vi "finding chrimson rails.vi"() -> ()   [LabVIEW 2014]
uses:
  <vilib>/userdefined/High Color/IMAQdx.ctl
  <vilib>/Utility/file.llb/Write To Spreadsheet File (DBL).vi
  <vilib>/vision/driver/NI_Vision_Acquisition_Software.lvlib
panel:
  in  "Tags":string
  out "Save Directory":path
  in  "Frames before Stimulus":i32
  out "Percent completed":dbl
  in  "Wait between stimuli (seconds)":dbl
  in  "pulse duration (frames)":i32
  in  "GO":bool
  in  "Array":dbl[](array[numeric])
  in  "Trials Per Voltage":i32
  in  "Frames":i32
  out "Error":string
  out "Buffer Number Out":u32
  out "Image":T1(plugin-control)
  in  "stop":bool
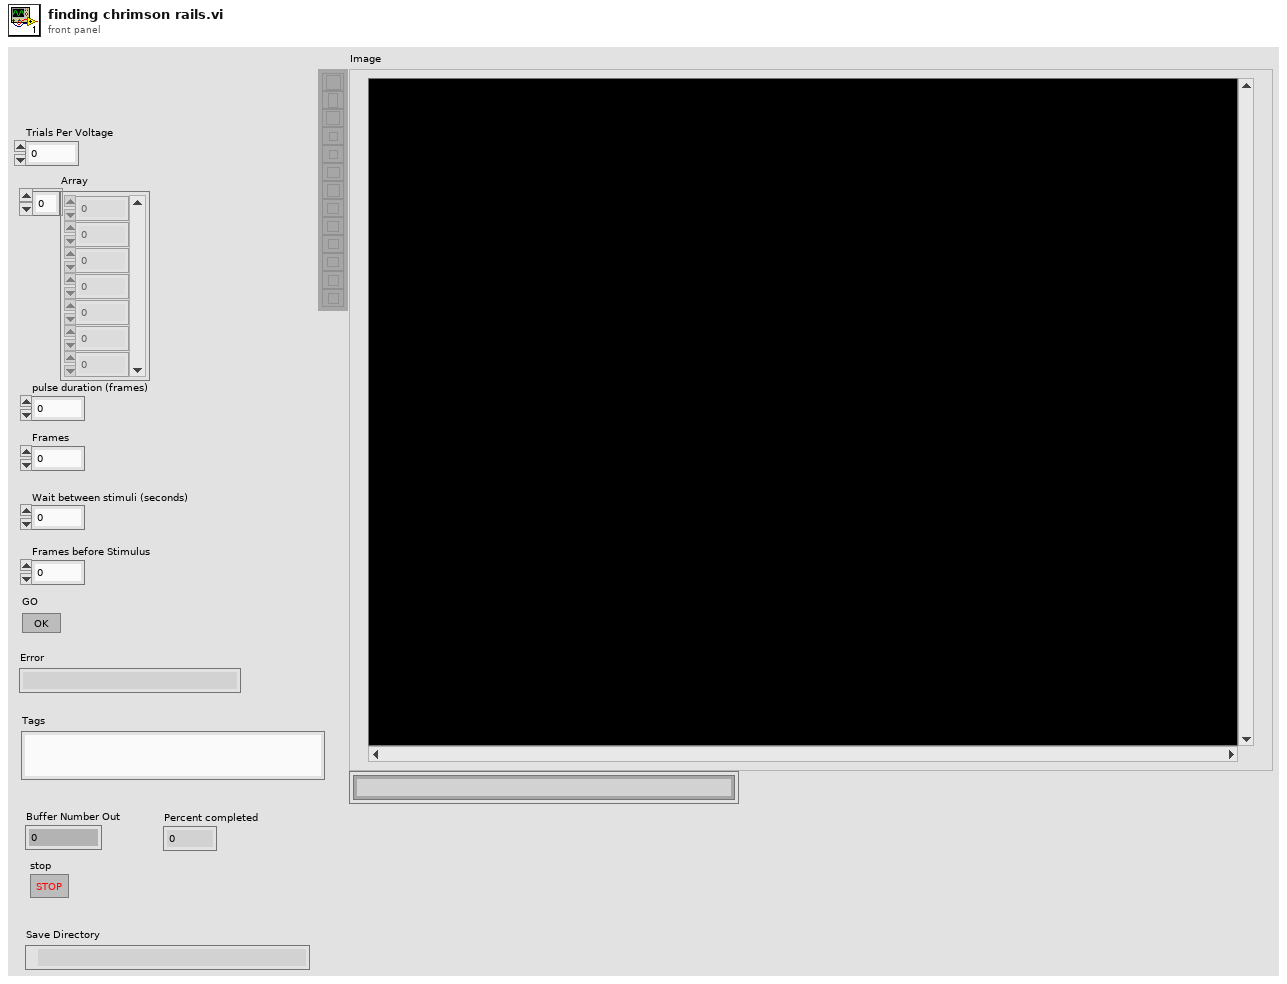
[diagram p1: front panel]
types:
  T1 = typedef "IMAQ Image.ctl" = refnum<image>
  T2 = typedef "IMAQdx.ctl" = refnum<k21>
  T3 = cluster{"Rows Per Strip":i32, "Photometric":i32, "Compression Type":i32}
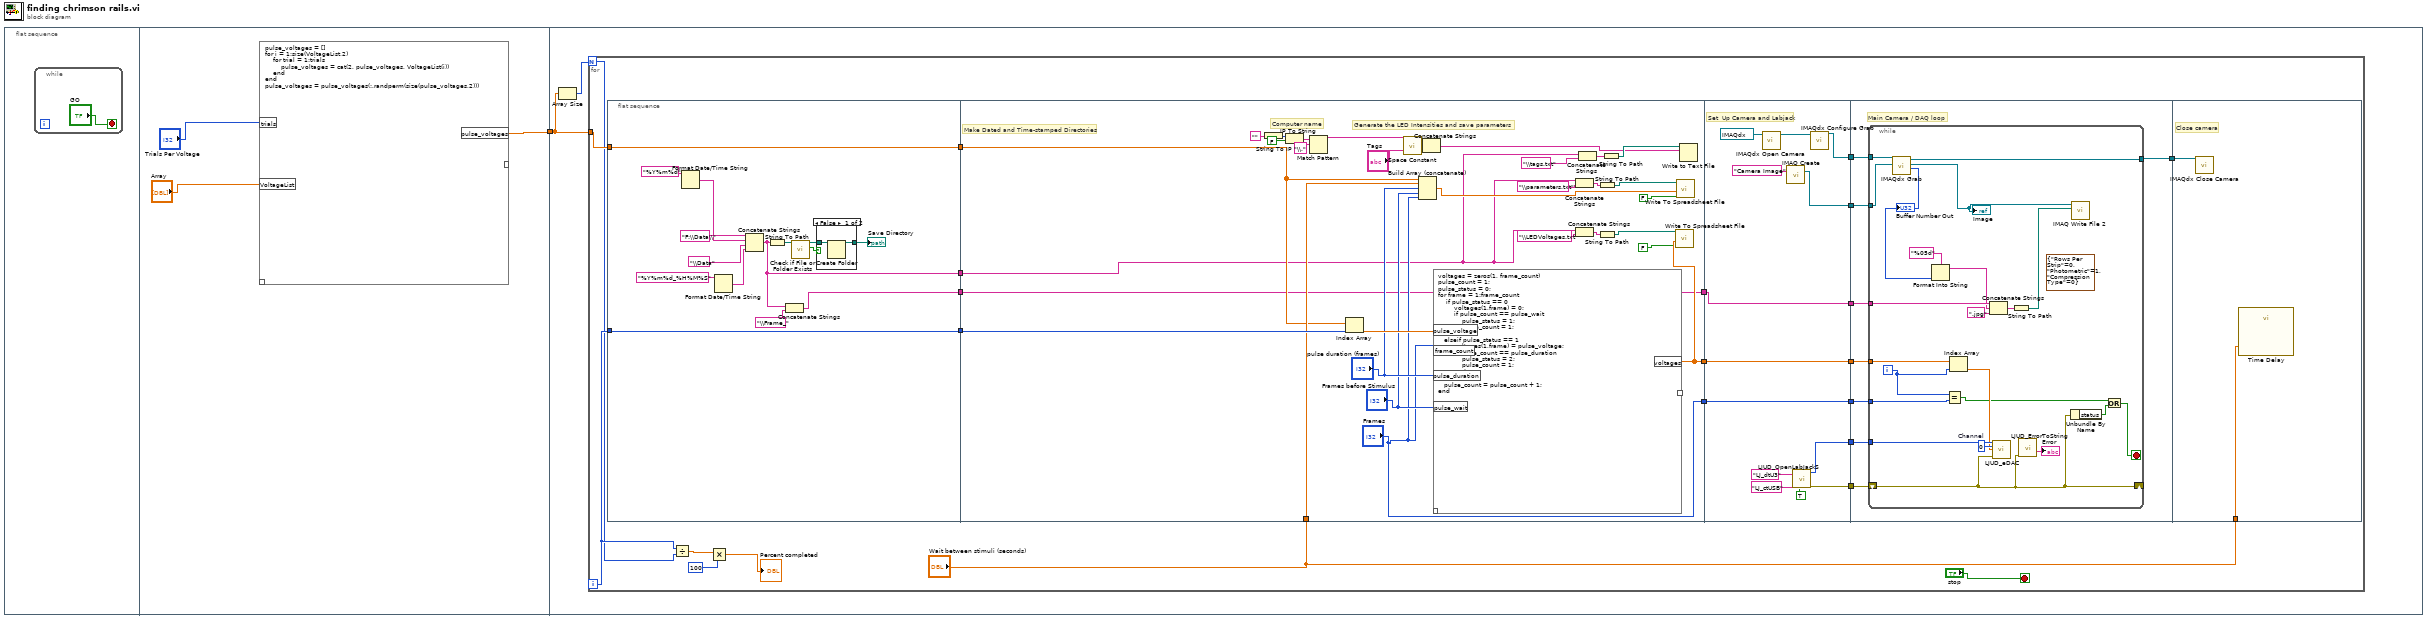
[diagram p0: block diagram]
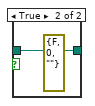
[diagram p2: hidden frame]
diagram:
  n1 = flat-sequence {
    tunnel: [w4] -> w1
    tunnel: w1 -> [w7]
    frame #0 {
      n2 = while {
        stop <- "GO" stop-if-true
      }
    }
    frame #1 {
      n3 = script code="pulse_voltages = []\nfor i = 1:size(VoltageList,2)\n    for trial = 1:trials\n        pulse_voltages = cat(2, pulse_voltages, VoltageList(i))\n    end\nend\npulse_voltages = pulse_voltages(:,randperm(size(pulse_voltages,2)))"("trials"="Trials Per Voltage", "VoltageList"="Array") -> ("pulse_voltages"=w4:dbl[])  [unwired: 1 in, 1 out]
    }
    frame #2 {
      n4 = Array Size(array=w7) -> (size(s)=w6:i32)
      n5 = for {
        N: w6 -> [w16]
        tunnel: w7 -> [w19]
        i -> [w17]
        stop <- "stop" stop-if-true
        n6 = flat-sequence {
          tunnel: w17 -> [w44]
          tunnel: w19 -> [w45]
          tunnel: [w45] -> w12
          tunnel: [w44] -> w11
          tunnel: [w32] -> w10
          tunnel: [w31] -> w9
          tunnel: [w62] -> w30
          tunnel: [w76] -> w29
          tunnel: ["Frames"] -> w28
          tunnel: "Wait between stimuli (seconds)" -> [w67]
          tunnel: w12 -> [w63]
          tunnel: w11 -> [w68]
          tunnel: w10 -> [w62]
          tunnel: w9 -> [w55]
          tunnel: w30 -> [w87]
          tunnel: [w89] -> w27
          tunnel: [w88] -> w26
          tunnel: [w87] -> w25
          tunnel: [w83] -> w24
          tunnel: [w82] -> w23
          tunnel: [w81] -> w22
          tunnel: w29 -> [w81]
          tunnel: w28 -> [w80]
          tunnel: [w80] -> w21
          tunnel: w27 -> [w100]
          tunnel: w26 -> [w99]
          tunnel: w25 -> [w98]
          tunnel: [w97] -> w20
          tunnel: w24 -> [w96]
          tunnel: w23 -> [w95]
          tunnel: w22 -> [w94]
          tunnel: w21 -> [w93]
          tunnel: w20 -> [w124]
          tunnel: "Wait between stimuli (seconds)" -> [w123]
          frame #0 {
            n7 = Format Date/Time String(time format string (%c)="%Y%m%d") -> (date/time string=w34:string)  [unwired: 2 in]
            n8 = Format Date/Time String(time format string (%c)="%Y%m%d_%H%M%S") -> (date/time string=w38:string)  [unwired: 2 in]
            n9 = Concatenate Strings("F:\\Data\\", w34, "\\Data", w38) -> (w31:string)
            n10 = String To Path(string=w31) -> (path=w37:path)
            n11 = Concatenate Strings(w31, "\\Frame_") -> (w32:string)
            n12 = call <vilib>:"Check if File or Folder Exists.vi"("path"=w37) -> ("file or folder exists?"=w42:bool, "dup path"=w41:path)  [unwired: 8 in, 1 out]
            n13 = case shown="False" w42 {
              tunnel: [w46 w48] -> w36
              tunnel: w41 -> [w47 w48]
              frame False {
                n14 = Create Folder(path (use dialog)=w47) -> (created path=w46:path)  [unwired: 2 in, 2 out]
              }
              frame True {
                (unwired) errorcluster {"status"=FALSE, "code"=0, "source"=""} ("error out")
              }
            }
            "Save Directory" <- w36
          }
          frame #1 {
            # "Computer name"
            # "Make Dated and Time-stamped Directories"
            # "Generate the LED Intensities and save parameters"
            n15 = String To IP(1:"") -> (0:w54:u32)
            n16 = IP To String(1:FALSE, 2:w54) -> (0:w51:string)
            n17 = Match Pattern(string=w51, regular expression="\\.") -> (before substring=w49:string)  [unwired: 1 in, 3 out]
            n18 = Index Array(array=w63, index=w68) -> (element=w69:dbl)
            n19 = call <vilib>:"Space Constant.vi"() -> ("String"=w57:string)
            n20 = Build Array (concatenate)(w63, w67, "pulse duration (frames)", "Frames before Stimulus", "Frames") -> (w70:dbl[])
            n21 = Concatenate Strings(w49, w57, "Tags") -> (w56:string)
            n22 = script code="voltages = zeros(1, frame_count)\npulse_count = 1;\npulse_status = 0;\nfor frame = 1:frame_count\n    if pulse_status == 0\n        voltages(1,frame) = 0;\n        if pulse_count == pulse_wait\n            pulse_status = 1;\n            pulse_count = 1;\n        end\n   elseif pulse_status == 1\n        voltages(1,frame) = pulse_voltage;\n        if pulse_count == pulse_duration\n            pulse_status = 2;\n            pulse_count = 1;\n        end\n   end\n   pulse_count = pulse_count + 1;\nend"("frame_count"="Frames", "pulse_voltage"=w69, "pulse_duration"="pulse duration (frames)", "pulse_wait"="Frames before Stimulus") -> ("voltages"=w76:dbl[])  [unwired: 1 in, 1 out]
            n23 = Concatenate Strings(w55, "\\LEDVoltages.txt") -> (w79:string)
            n24 = Concatenate Strings(w55, "\\parameters.txt") -> (w74:string)
            n25 = Concatenate Strings(w55, "\\tags.txt") -> (w60:string)
            n26 = String To Path(string=w79) -> (path=w78:path)
            n27 = String To Path(string=w74) -> (path=w73:path)
            n28 = String To Path(string=w60) -> (path=w59:path)
            n29 = call-poly <vilib>:"Write To Spreadsheet File.vi"("append to file? (new file:F)"=FALSE, "1D data"=w76, "file path (dialog if empty)"=w78) -> ()  [unwired: 5 in, 1 out]
            n30 = call-poly <vilib>:"Write To Spreadsheet File.vi"("append to file? (new file:F)"=FALSE, "1D data"=w70, "file path (dialog if empty)"=w73) -> ()  [unwired: 5 in, 1 out]
            n31 = Write to Text File(file (use dialog)=w59, text=w56) -> ()  [unwired: 2 in, 3 out]
          }
          frame #2 {
            # "Set  Up Camera and Labjack"
            n32 = call <vilib>:"IMAQdx Open Camera.vi"("Session In"=T2 "cam0") -> ("Session Out"=w91:T2)  [unwired: 9 in, 1 out]
            n33 = call "IMAQ Create"("Image Name"="Camera Image") -> ("New Image"=w88:T1)  [unwired: 4 in, 1 out]
            n34 = call "LJUD_OpenLabJackS.vi"("FirstFound"=TRUE, "ConnectionType"="LJ_ctUSB", "DeviceType"="LJ_dtU3") -> ("error out"=w82:errorcluster, "Handle"=w83:i32)  [unwired: 6 in, 1 out]
            n35 = call <vilib>:"IMAQdx Configure Grab.vi"("Session In"=w91) -> ("Session Out"=w89:T2)  [unwired: 9 in, 1 out]
          }
          frame #3 {
            # "Main Camera / DAQ loop"
            n36 = while {
              tunnel: w100 -> [w122]
              tunnel: [w121] -> w97
              tunnel: w99 -> [w120]
              tunnel: w98 -> [w118]
              tunnel: w96 -> [w111]
              shift-right: [w110] -> _
              shift-left: w95 -> [w110]
              tunnel: w94 -> [w103]
              tunnel: w93 -> [w102]
              i -> [w104]
              stop <- w101 stop-if-true
              w109 = 0  # Channel
              (unwired) T3 {"Rows Per Strip"=0, "Photometric"=1, "Compression Type"=0} ("TIFF Options")
              n37 = call <vilib>:"IMAQdx Grab.vi"("Image In"=w120, "Session In"=w122) -> ("Buffer Number Out"=w114:u32, "Image Out"=w119:T1, "Session Out"=w121:T2)  [unwired: 6 in, 1 out]
              "Image" <- w119
              "Buffer Number Out" <- w114
              n38 = Format Into String(format string="%05d" ("string"), w114) -> (resulting string=w113:string)  [unwired: 2 in, 1 out]
              n39 = Equal?(x=w104, y=w102) -> (x = y?=w105:bool)
              n40 = Index Array(array=w103, index=w104) -> (element=w107:dbl)
              n41 = Concatenate Strings(w118, w113, ".jpg" ("string")) -> (w116:string)
              n42 = call "LJUD_eDAC.vi"("Handle In"=w111, "Channel"=w109, "Voltage"=w107, "error in"=w110) -> ()  [unwired: 10 in, 2 out]
              n43 = String To Path(string=w116) -> (path=w115:path)
              n44 = call "LJUD_ErrorToString.vi"("error in"=w110) -> ("String"=→"Error":string)  [unwired: 10 in]
              n45 = Unbundle By Name(w110) -> ("status"=w106:bool)
              n46 = call-poly "IMAQ Write File 2"("File Path"=w115, "Image"=w119) -> ()  [unwired: 8 in, 2 out]
              n47 = Or(x=w105, y=w106) -> (x .or. y?=w101:bool)
            }
          }
          frame #4 {
            # "Close camera"
            n48 = call <vilib>:"IMAQdx Close Camera.vi"("Session In"=w124) -> ()  [unwired: 10 in, 1 out]
            n49 = call "Time Delay"("Delay Time (s)"=w123) -> ()  [unwired: 10 in, 1 out]
          }
        }
        n50 = Divide(x=w17, y=w16) -> (x/y=w15:dbl)
        n51 = Multiply(x=w15, y=100) -> (x*y=→"Percent completed":dbl)
      }
    }
  }
